vi "Read MODBUS Serial Parameters.vi"(8 "error in (no error)":errorcluster, 11 "MODBUS in":refnum<class "MODBUS.lvclass">) -> (0 "error out":errorcluster, 2 "MODBUS Serial Parameters":T1={"Mode"=enum."RTU", "Default Slave Address"=111, "MODBUS timeout"=1000, "Baud Rate"=38400, "Parity"=0, "Flow Control"=0} {"Flow Control" items=["None", "XON/XOFF", "RTS/CTS", "XON/XOFF & RTS/CTS", "DTR/DSR", "XON/XOFF & DTR/DSR"]; "Parity" items=["None", "Odd", "Even", "Mark", "Space"]}, 3 "MODBUS out":refnum<class "MODBUS.lvclass">)   [LabVIEW 2016, in "MODBUS.lvclass"]
uses:
  MODBUS.lvclass
  MODBUS parameters type.ctl
  MODBUS.lvclass/MODBUS.ctl
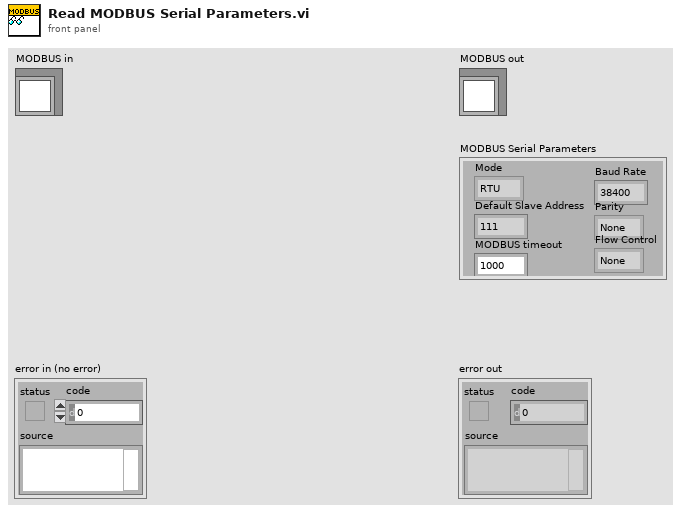
[diagram p1: front panel]
types:
  T1 = typedef "MODBUS parameters type.ctl" = cluster{"Mode":enum16{"RTU", "ASCII"}, "Default Slave Address":u8, "MODBUS timeout":u32, "Baud Rate":u32, "Parity":u16, "Flow Control":u16}
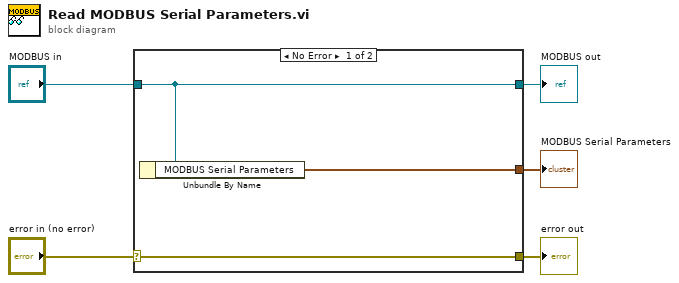
[diagram p0: block diagram]
diagram:
  n1 = case shown="No Error" "error in (no error)" {
    selector: "error in (no error)" -> [w8 w9]
    tunnel: [w8 w9] -> w4
    tunnel: [w7 w10] -> w2
    tunnel: "MODBUS in" -> [w7 w10]
    tunnel: [w6 _] -> w1
    frame No Error {
      n2 = Unbundle By Name(w7) -> ("MODBUS Serial Parameters"=w6:T1)
    }
    frame Error {
    }
  }
  "error out" <- w4
  "MODBUS out" <- w2
  "MODBUS Serial Parameters" <- w1
